vi "Reset and Read.vi"(8 "error in (no error)":errorcluster, 9 "SL voltage (V)":dbl, 10 "WL voltage (V)":dbl, 11 "IVI Refnum in":refnum<k15>) -> (0 "error out":errorcluster, 1 "Current (A)":dbl, 2 "Resistance (ohm)":dbl, 3 "IVI Refnum out":refnum<k15>)   [LabVIEW 2018]
uses:
  <instrlib>/niDigital/niDigital.llb/niDigital Burst Pattern (Burst Only).vi
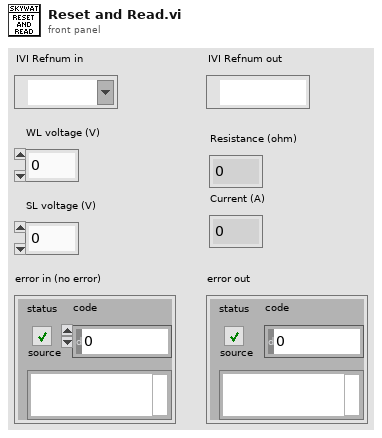
[diagram p1: front panel]
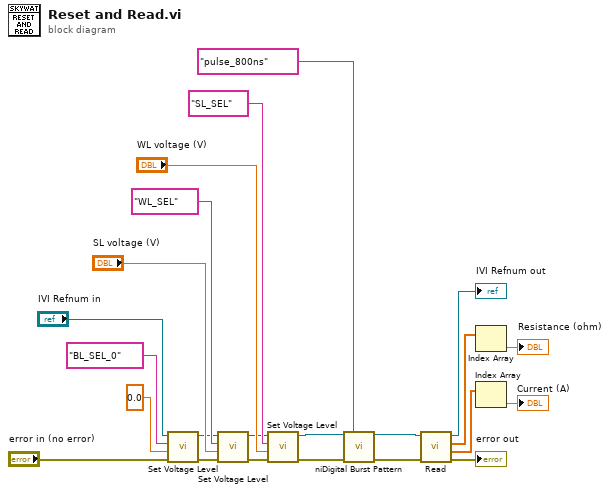
[diagram p0: block diagram]
diagram:
  n1 = call "Set Voltage Level.vi"("error in (no error)"="error in (no error)", "level (V)"=0.0, "channel list"="BL_SEL_0", "instrument handle"="IVI Refnum in") -> ("error out"=w7:errorcluster, "instrument handle out"=w6:refnum<k15>)  [unwired: 6 in]
  n2 = call "Set Voltage Level.vi"("error in (no error)"=w7, "level (V)"="SL voltage (V)", "channel list"="WL_SEL", "instrument handle"=w6) -> ("error out"=w4:errorcluster, "instrument handle out"=w5:refnum<k15>)  [unwired: 6 in]
  n3 = call "Set Voltage Level.vi"("error in (no error)"=w4, "level (V)"="WL voltage (V)", "channel list"="SL_SEL", "instrument handle"=w5) -> ("error out"=w15:errorcluster, "instrument handle out"=w16:refnum<k15>)  [unwired: 6 in]
  n4 = call-poly <instrlib>:"niDigital Burst Pattern.vi"("instrument handle"=w16, "start label"="pulse_800ns", "error in"=w15) -> ("instrument handle out"=w18:refnum<k15>, "error out"=w17:errorcluster)  [unwired: 11 in]
  n5 = call "Read.vi"("error in (no error)"=w17, "instrument handle"=w18) -> ("error out"=→"error out":errorcluster, "currents (A)"=w2:dbl[], "resistances (ohm)"=w19:dbl[], "instrument handle out"=→"IVI Refnum out":refnum<k15>)  [unwired: 6 in]
  n6 = Index Array(array=w19) -> (element=→"Resistance (ohm)":dbl)  [unwired: 1 in]
  n7 = Index Array(array=w2) -> (element=→"Current (A)":dbl)  [unwired: 1 in]
